vi "Pick HDI.vi"(8 "error in":errorcluster, 9 "Slot":i32, 10 "Chuck":i32, 11 "PickerTool in":refnum<class "PickerTool Class.lvclass">) -> (0 "error out":errorcluster, 3 "PickerTool out":refnum<class "PickerTool Class.lvclass">)   [LabVIEW 2017, in "PickerTool Class.lvclass"]
uses:
  PickerTool Class.lvclass
  Vec3d Class/Vec3d Class.lvclass
  WorkTable Class/WorkTable Class.lvclass
  Config Manager Class/Type Definitions/Offset.ctl
  Config Manager Class/Type Definitions/Part Type.ctl
  FlexWorktable/FlexWorktable.lvclass
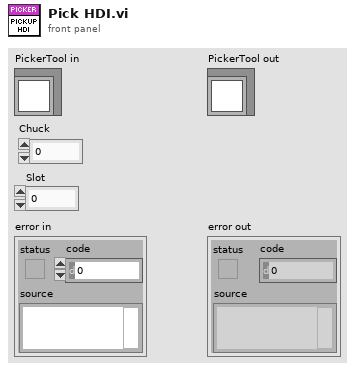
[diagram p1: front panel]
types:
  T1 = enum16{"Empty", "Bare HDI", "Unglued", "Stamped", "PartOnTop", "Weighted", "Unpotted", "Potted"}
  T2 = typedef "Part Type.ctl" = enum16{"BBM", "HDI", "BARE HDI", "GLUERESERVOIR", "STAMP_1", "STAMP_2", "STAMP_3", "STAMP_4", "STAMP_5", "STAMP_6", "STAMP_7", "STAMP_8", "WEIGHT_1", "WEIGHT_2", "WEIGHT_3", "WEIGHT_4", "WEIGHT_5", "WEIGHT_6", "WEIGHT_7", "WEIGHT_8", "WEIGHT_9", "WEIGHT_10", "WEIGHT_11", "WEIGHT_12", "WEIGHT_13", "WEIGHT_14", "WEIGHT_15", "WEIGHT_16", "PICKER_TOOL", "GRABER_TOOL", "TFPX_HDI_V2"}
  T3 = typedef "Offset.ctl" = enum16{"tool_holder_offset"}
  T4 = typedef "Worktable_Module Slot.ctl" = cluster{"Slot State":enum16{"Empty", "Bare HDI", "Unglued", "Stamped", "PartOnTop", "Weighted", "Unpotted", "Potted"}, "BBM Type":enum16{"None", "BBM", "GlassSlide"}, "HDI Type":enum16{"None", "HDI", "Polyimide"}, "Vacuum Channel":u8, "Location/Orientation BBM":T5, "Location/Orientation HDI":T5, "S/N":string}
  T5 = typedef "Position_Orientation.ctl" = cluster{"Center":refnum<class "Vec3d Class.lvclass">, "Orientation":refnum<class "Orient3d Class.lvclass">}
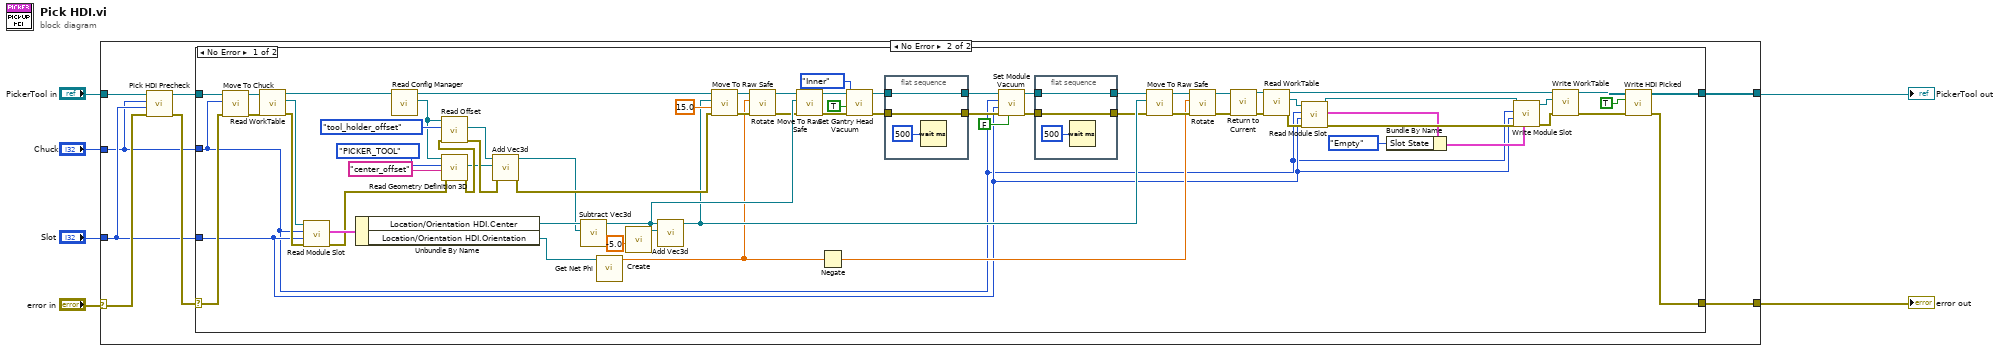
[diagram p0: block diagram]
diagram:
  n1 = case shown="No Error" "error in" {
    selector: "error in" -> [w7 w15]
    tunnel: [w7 w14] -> w5
    tunnel: [w8 w13] -> w3
    tunnel: "PickerTool in" -> [w8 w16]
    tunnel: "Slot" -> [_ w10]
    tunnel: "Chuck" -> [_ w9]
    frame Error {
    }
    frame No Error {
      n2 = call "Pick HDI Precheck.vi"("error in"=w15, "Slot Number in"=w10, "Chuck Number in"=w9, "PickupTool Class in"=w16) -> ("error out"=w11:errorcluster, "PickupTool Class out"=w12:refnum<class "PickerTool Class.lvclass">)  [unwired: 6 in]
      n3 = case shown="No Error" w11 {
        selector: w11 -> [w84 w93]
        tunnel: [w17 w93] -> w14
        tunnel: w12 -> [w85 w92]
        tunnel: [w21 w92] -> w13
        tunnel: w10 -> [w24 _]
        tunnel: w9 -> [w23 _]
        frame No Error {
          n4 = call-dynamic "Move To Chuck.vi"("error in"=w84, "Chuck"=w23, "Gantry in"=w85) -> ("error out"=w73:errorcluster, "Gantry out"=w77:refnum<class "PickerTool Class.lvclass">)  [unwired: 7 in]
          n5 = call-dynamic "Read WorkTable.vi"("error in"=w73, "Gantry Class in"=w77) -> ("error out"=w82:errorcluster, "Worktable"=w83:refnum<class "FlexWorktable.lvclass">, "Gantry Class out"=w76:refnum<class "PickerTool Class.lvclass">)  [unwired: 7 in]
          n6 = call-dynamic "Read Module Slot.vi"("error in"=w82, "slot"=w24, "chuck"=w23, "WorkTable in"=w83) -> ("error out"=w71:errorcluster, "Module Slot"=w81:T4)  [unwired: 5 in, 1 out]
          n7 = Unbundle By Name(w81) -> ("Location/Orientation HDI.Center"=w67:refnum<class "Vec3d Class.lvclass">, "Location/Orientation HDI.Orientation"=w57:refnum<class "Orient3d Class.lvclass">)
          n8 = call-dynamic "Read Config Manager.vi"("Gantry in"=w76) -> ("Config Manager"=w72:refnum<class "Config Manager Class.lvclass">, "Gantry out"=w75:refnum<class "PickerTool Class.lvclass">)  [unwired: 8 in, 1 out]
          n9 = call "Read Geometry Definition 3D.vi"("error in"=w71, "Feature"="center_offset", "Part Type"=Part_Type."PICKER_TOOL", "Config Manager in"=w72) -> ("error out"=w70:errorcluster, "Feature Coordinates"=w68:refnum<class "Vec3d Class.lvclass">)  [unwired: 5 in, 1 out]
          n10 = call "Read Offset.vi"("error in"=w70, "Offset"=Offset."tool_holder_offset", "Config Manager in"=w72) -> ("error out"=w69:errorcluster, "Vec3d out"=w80:refnum<class "Vec3d Class.lvclass">)  [unwired: 6 in, 1 out]
          n11 = call-dynamic "Add Vec3d.vi"("error in (no error)"=w69, 10:"Vec3d Class in"=w68, 11:"Vec3d Class in"=w80) -> ("error out"=w78:errorcluster, "Vec3d Class out"=w66:refnum<class "Vec3d Class.lvclass">)  [unwired: 7 in]
          n12 = call "Subtract Vec3d.vi"("Vec3d in 2"=w66, "Vec3d in 1"=w67) -> ("Vec3d Class out"=w63:refnum<class "Vec3d Class.lvclass">)  [unwired: 8 in, 1 out]
          n13 = call "Get Net Phi.vi"("Orient3d"=w57) -> ("phi(deg)"=w36:dbl)  [unwired: 8 in, 2 out]
          n14 = call "Create.vi"("Z"=-5.0) -> ("Vec3d Class out"=w64:refnum<class "Vec3d Class.lvclass">)  [unwired: 9 in, 1 out]
          n15 = call-dynamic "Add Vec3d.vi"(10:"Vec3d Class in"=w64, 11:"Vec3d Class in"=w63) -> ("Vec3d Class out"=w58:refnum<class "Vec3d Class.lvclass">)  [unwired: 8 in, 1 out]
          n16 = call-dynamic "Move To Raw Safe.vi"("error in"=w78, "Speed(mm/s)"=15.0 ("Speed"), "Destination"=w58, "Gantry in"=w75) -> ("error out"=w54:errorcluster, "Gantry out"=w56:refnum<class "PickerTool Class.lvclass">)  [unwired: 6 in]
          n17 = call-dynamic "Rotate.vi"("error in"=w54, "distance(deg)"=w36, "Gantry in"=w56) -> ("error out"=w53:errorcluster, "Gantry out"=w55:refnum<class "PickerTool Class.lvclass">)  [unwired: 7 in]
          n18 = call-dynamic "Move To Raw Safe.vi"("error in"=w53, "Destination"=w63, "Gantry in"=w55) -> ("error out"=w61:errorcluster, "Gantry out"=w62:refnum<class "PickerTool Class.lvclass">)  [unwired: 7 in]
          n19 = Negate(x=w36) -> (-x=w48:dbl)
          n20 = call-dynamic "Set Gantry Head Vacuum.vi"("error in (no error)"=w61, "On/Off"=TRUE, "Inner/Outer"=enum16{"Outer", "Inner"}."Inner", "Gantry Class in"=w62) -> ("error out"=w41:errorcluster, "Gantry Class out"=w42:refnum<class "PickerTool Class.lvclass">)  [unwired: 6 in]
          n21 = flat-sequence {
            tunnel: w42 -> [w88]
            tunnel: [w88] -> w40
            tunnel: w41 -> [w87]
            tunnel: [w87] -> w39
            frame #0 {
              n22 = Wait (ms)(milliseconds to wait=u32 500) -> ()  [unwired: 1 out]
            }
          }
          n23 = call-dynamic "Set Module Vacuum.vi"("On/Off"=FALSE, "error in"=w39, "Slot Number"=w24, "Chuck Number"=w23, "Gantry in"=w40) -> ("error out"=w45:errorcluster, "Gantry out"=w46:refnum<class "PickerTool Class.lvclass">)  [unwired: 5 in]
          n24 = flat-sequence {
            tunnel: w46 -> [w91]
            tunnel: [w91] -> w44
            tunnel: w45 -> [w90]
            tunnel: [w90] -> w43
            frame #0 {
              n25 = Wait (ms)(milliseconds to wait=u32 500) -> ()  [unwired: 1 out]
            }
          }
          n26 = call-dynamic "Move To Raw Safe.vi"("error in"=w43, "Destination"=w58, "Gantry in"=w44) -> ("error out"=w50:errorcluster, "Gantry out"=w52:refnum<class "PickerTool Class.lvclass">)  [unwired: 7 in]
          n27 = call-dynamic "Rotate.vi"("error in"=w50, "distance(deg)"=w48, "Gantry in"=w52) -> ("error out"=w49:errorcluster, "Gantry out"=w51:refnum<class "PickerTool Class.lvclass">)  [unwired: 7 in]
          n28 = call-dynamic "Return to Current.vi"("error in"=w49, "Gantry in"=w51) -> ("error out"=w25:errorcluster, "Gantry out"=w26:refnum<class "PickerTool Class.lvclass">)  [unwired: 8 in]
          n29 = call-dynamic "Read WorkTable.vi"("error in"=w25, "Gantry Class in"=w26) -> ("error out"=w30:errorcluster, "Worktable"=w35:refnum<class "FlexWorktable.lvclass">, "Gantry Class out"=w34:refnum<class "PickerTool Class.lvclass">)  [unwired: 7 in]
          n30 = call-dynamic "Read Module Slot.vi"("error in"=w30, "slot"=w24, "chuck"=w23, "WorkTable in"=w35) -> ("error out"=w31:errorcluster, "Module Slot"=w28:T4, "WorkTable out"=w29:refnum<class "WorkTable Class.lvclass">)  [unwired: 5 in]
          n31 = Bundle By Name(cluster=w28, "Slot State"=T1."Empty") -> (w27:T4)
          n32 = call-dynamic "Write Module Slot.vi"("Module Slot"=w27, "error in"=w31, "slot"=w24, "chuck"=w23, "WorkTable in"=w29) -> ("error out"=w32:errorcluster, "WorkTable out"=w33:refnum<class "WorkTable Class.lvclass">)  [unwired: 5 in]
          n33 = call-dynamic "Write WorkTable.vi"("error in (no error)"=w32, "FlexWorktable"=w33, "Gantry Class in"=w34) -> ("error out"=w18:errorcluster, "Gantry Class out"=w19:refnum<class "PickerTool Class.lvclass">)  [unwired: 7 in]
          n34 = call "Write HDI Picked.vi"("error in (no error)"=w18, "HDI Picked"=TRUE, "PickerTool Class in"=w19) -> ("error out"=w17:errorcluster, "PickerTool Class out"=w21:refnum<class "PickerTool Class.lvclass">)  [unwired: 7 in]
        }
        frame Error {
        }
      }
    }
  }
  "error out" <- w5
  "PickerTool out" <- w3
